vi "saveData.vi"(5 "파일명":string, 8 "error in":errorcluster caption="에러 입력", 10 "데이터":string, 11 "기능":T1) -> (0 "error out":errorcluster caption="에러 출력", 2 "데이터용량(byte)":i64, 3 "데이터개수":i32)   [LabVIEW 2018]
uses:
  control/enumBaseFunction.ctl
  <vilib>/Utility/sysdir.llb/System Directory Type.ctl
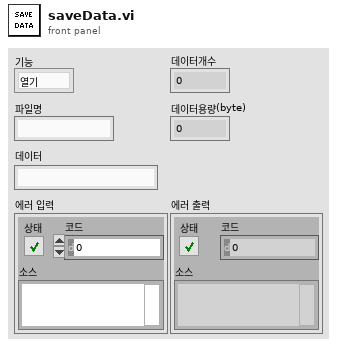
[diagram p1: front panel]
types:
  T1 = typedef "enumBaseFunction.ctl" = enum16{"열기", "쓰기", "확인", "닫기"}
  T2 = enum16{"open", "replace", "create", "open or create", "replace or create", "replace or create with confirmation"}
  T3 = typedef "System Directory Type.ctl" = i32
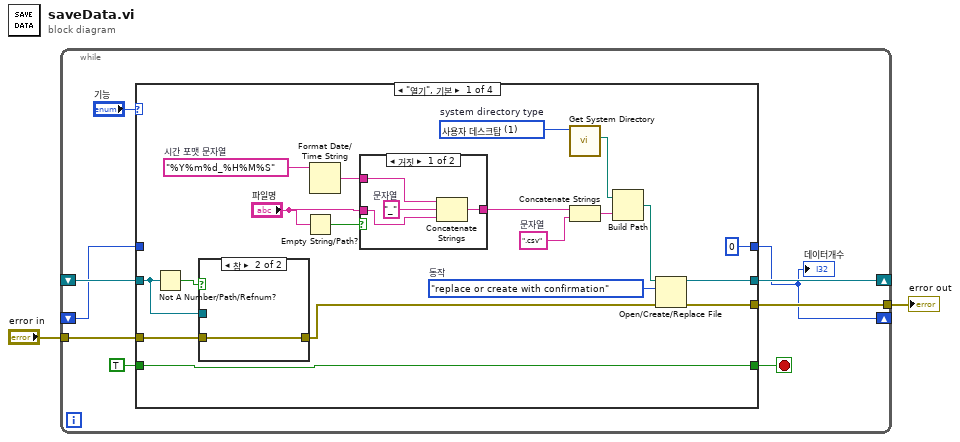
[diagram p0: block diagram]
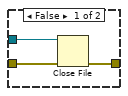
[diagram p2: hidden frame]
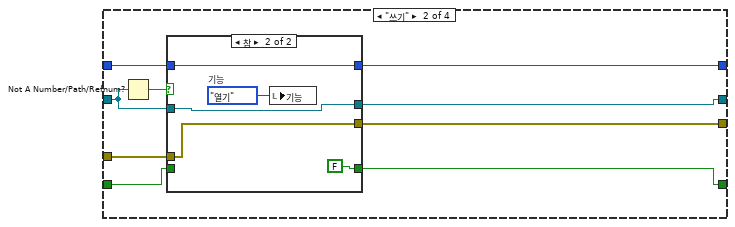
[diagram p4: hidden frame]
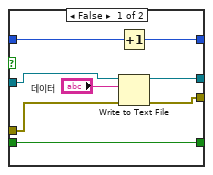
[diagram p5: hidden frame]
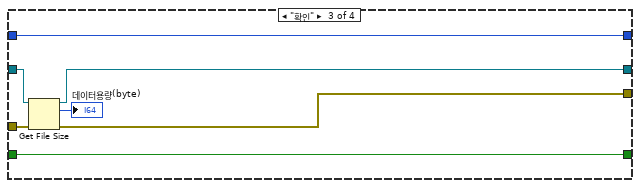
[diagram p6: hidden frame]
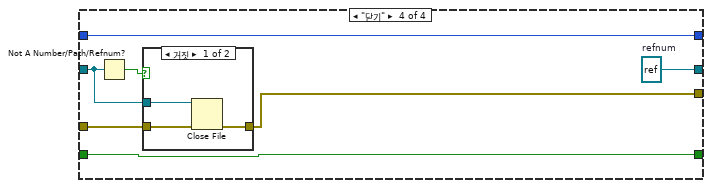
[diagram p7: hidden frame]
diagram:
  n1 = while {
    shift-right: [w11] -> _
    shift-left: _ -> [w10]
    tunnel: "error in" -> [w9]
    tunnel: [w8] -> w1
    shift-right: [w5] -> _
    shift-left: _ -> [w6]
    stop <- w4 stop-if-true
    n2 = case shown="\"열기\", 기본" "기능" {
      tunnel: [w23 w48 w63 w73] -> w11
      tunnel: w10 -> [w17 w43 w68 w70]
      tunnel: w9 -> [w15 w46 w67 w75]
      tunnel: [w22 w47 w66 w74] -> w8
      tunnel: w6 -> [_ w45 w64 w72]
      tunnel: [0 w44 w64 w72] -> w5
      tunnel: [w20 w41 w62 w71] -> w4
      tunnel: TRUE -> [w20 w40 w62 w71]
      frame "열기", Default {
        w12 = ".csv"  # 문자열
        w19 = T2."replace or create with confirmation"  # 동작
        w26 = "%Y%m%d_%H%M%S"  # 시간 포맷 문자열
        w25 = T3 1 items=["사용자 홈"=0, "사용자 데스크탑"=1, "사용자 문서"=2, "사용자 어플리케이션 데이터"=3, "사용자 환경"=4, "사용자 임시"=5, "퍼블릭 문서"=6, "퍼블릭 어플리케이션 데이터"=7, "퍼블릭 환경"=8, "퍼블릭 캐시"=13, "시스템 코어 라이브러리"=9, "시스템 설치된 라이브러리"=10, "어플리케이션 파일"=11, "부팅 볼륨 루트"=12]  # system directory type
        n3 = Not A Number/Path/Refnum?(number/path/refnum=w17) -> (NaN/Path/Refnum?=w18:bool)
        n4 = case shown="참" w18 {
          tunnel: w17 -> [w33 _]
          tunnel: w15 -> [w32 w34]
          tunnel: [w31 w34] -> w16
          frame False {
            n5 = Close File(refnum=w33, error in=w32) -> (error out=w31:errorcluster)  [unwired: 1 out]
          }
          frame True {
          }
        }
        n6 = Empty String/Path?(string/path="파일명") -> (empty?=w29:bool)
        n7 = Format Date/Time String(time format string (%c)=w26) -> (date/time string=w28:string)  [unwired: 2 in]
        n8 = case shown="거짓" w29 {
          tunnel: [w35 w39] -> w14
          tunnel: w28 -> [w38 w39]
          tunnel: "파일명" -> [w36 _]
          frame False {
            w37 = "_"  # 문자열
            n9 = Concatenate Strings(w38, w37, w36) -> (w35:string)
          }
          frame True {
          }
        }
        n10 = call <vilib>:"Get System Directory.vi"("system directory type"=w25) -> ("system directory"=w30:path)  [unwired: 10 in]
        n11 = Concatenate Strings(w14, w12) -> (w13:string)
        n12 = Build Path(base path=w30, name or relative path=w13) -> (appended path=w24:path)
        n13 = Open/Create/Replace File(file path (use dialog)=w24, error in=w16, operation (0:open)=w19) -> (refnum out=w23:refnum<file>, error out=w22:errorcluster)  [unwired: 3 in, 1 out]
      }
      frame "쓰기" {
        n14 = Not A Number/Path/Refnum?(number/path/refnum=w43) -> (NaN/Path/Refnum?=w42:bool)
        n15 = case shown="참" w42 {
          tunnel: w43 -> [w56 w60]
          tunnel: [w55 w60] -> w48
          tunnel: [w54 w59] -> w47
          tunnel: w46 -> [w53 w59]
          tunnel: w45 -> [w51 w58]
          tunnel: [w50 w58] -> w44
          tunnel: [w49 FALSE] -> w41
          tunnel: w40 -> [w49 _]
          frame False {
            n16 = Increment(x=w51) -> (x+1=w50:i32)
            n17 = Write to Text File(file (use dialog)=w56, text="데이터", error in=w53) -> (refnum out=w55:refnum<file>, error out=w54:errorcluster)  [unwired: 1 in, 1 out]
          }
          frame True {
            w61 = enumBaseFunction."열기"  # 기능
            n18 = local write "기능"(w61) -> ()
          }
        }
      }
      frame "확인" {
        n19 = Get File Size(file=w68, error in=w67) -> (refnum out=w63:refnum<file>, size (in bytes)=→"데이터용량(byte)":i64, 0:w66:errorcluster)
      }
      frame "닫기" {
        w73 = refnum<file> refnum  # refnum
        n20 = Not A Number/Path/Refnum?(number/path/refnum=w70) -> (NaN/Path/Refnum?=w69:bool)
        n21 = case shown="거짓" w69 {
          tunnel: w70 -> [w78 _]
          tunnel: w75 -> [w77 w79]
          tunnel: [w76 w79] -> w74
          frame False {
            n22 = Close File(refnum=w78, error in=w77) -> (error out=w76:errorcluster)  [unwired: 1 out]
          }
          frame True {
          }
        }
      }
    }
    "데이터개수" <- w5
  }
  "error out" <- w1
